vi "UI_SettingsUpdate.vi"(8 "error in (no error)":errorcluster) -> (0 "error out":errorcluster)   [LabVIEW 2020]
uses:
  Global Variables/gl_UI Ctrl Refs.vi
  Globals/gl_Calibration globals.vi
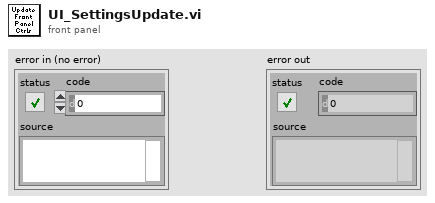
[diagram p1: front panel]
types:
  T1 = typedef "General Scan Parameters.ctl" = cluster{"Field of View":sgl, "Frame Size":u16, "Dwell Time (ms)":dbl, "Wavelength (nm)":dbl, "Zoom":dbl, "AOL Xc":sgl, "AOL Yc":sgl, "AOL Zc":sgl, "AOL Mode":enum16{"Raster", "Structural", "Pointing", "Mini Scan", "Alignment"}, "Imaging Mode":enum16{"Live Imaging", "AOL Zstack", "Motor Zstack", "Functional Imaging"}}
  T2 = typedef "UI ctrl refs cluster.ctl" = cluster{"Top level VI path":path, "Top level VI ref":refnum<vi>, "User menu ref":refnum<k9>, "Sub Panel control":refnum<vi>, "Imaging Param Tab":refnum<vi>, "Occurrence-Start drivers":refnum<k4>, "Occurrence-Speed logging initialised":refnum<k4>, "Occurrence-XYZ stage initialised":refnum<k4>, "Exit button":refnum<vi>, "Status ind":refnum<vi>, "Set as origin":refnum<vi>, "Speed Logging":refnum<vi>, "Time Lapse":refnum<vi>, "Live Imaging":refnum<vi>, "AOL Z Stack":refnum<vi>, "Motor Z Stack":refnum<vi>, "Funct Acq button":refnum<vi>, "Hard Shutter":refnum<vi>, "Virtual Shutter":refnum<vi>, "Laser Power":refnum<vi>, "AOL Mode":refnum<vi>, "Frame Size":refnum<vi>, "Field of View":refnum<vi>, "Dwell Time":refnum<vi>, "Zoom":refnum<vi>, "AOL Z":refnum<vi>, "Objective":refnum<vi>, "Axis":refnum<vi>, "Paths & Names":refnum<vi>, "Experiment folder path (ind.)":refnum<vi>, "Last State (Ind.)":refnum<vi>, "Averages":refnum<vi>, "Angle (degrees)":refnum<vi>, "X centre":refnum<vi>, "Y centre":refnum<vi>, "Plane Mode":refnum<vi>, "# Planes":refnum<vi>, "Z Start":refnum<vi>, "Z Stop":refnum<vi>, "Z Step":refnum<vi>, "PMT 1":refnum<vi>, "PMT 2":refnum<vi>, "Stage XYZ Position":refnum<vi>, "Pockels@Z Start":refnum<vi>, "Pockels@Z Stop":refnum<vi>, "Obtain Z Start":refnum<vi>, "Obtain Z Stop":refnum<vi>, "Live stim.trig.period":refnum<vi>, "Live stim.trig.enable":refnum<vi>, "Movement Correction":refnum<vi>, "Load Reference Image":refnum<vi>, "XY Stage Move":refnum<vi>, "MovCor Cluster":refnum<vi>, "RefDAQParam":refnum<vi>, "Funct. Acq. Pockels Modulation":refnum<vi>, "Ref Laser Power":refnum<vi>, "Enable Video Recording":refnum<vi>, "Video Record-Live Imaging":refnum<vi>, "Video Record-Funct acq":refnum<vi>, "Reference Source":refnum<vi>, "AOL Z-stack Chirps Ready (ind)":refnum<vi>, "Target time between mov.cor. ref triggers (ms)":refnum<vi>, "Funct. Acq. Ref frame save":refnum<vi>, "Tracking button":refnum<vi>, "Show ref plots window":refnum<vi>, "Center freq ind (nm)":refnum<vi>, "Pickup mode (ind)":refnum<vi>, "Logging queue (ind)":refnum<vi>, "Back aperture power (ind.)":refnum<vi>, "Power after objective (ind.)":refnum<vi>, "Switch user":refnum<vi>, "Ls1 Conn. Status":refnum<vi>, "Ls1Tuning Status":refnum<vi>, "Ls1 Faults":refnum<vi>, "Ls1 Connection":refnum<vi>, "Ls1 Mode":refnum<vi>, "Ls1 POWER [mW]":refnum<vi>, "Ls1Shutter":refnum<vi>, "Ls1 Wavelength":refnum<vi>, "Ls1 Note":refnum<vi>, "Ls1 Confirm Wav":refnum<vi>, "Ls1 PreChrp Prism1":refnum<vi>, "Ls1 PreChrp Prism2":refnum<vi>, "Ls1 wav top Ind":refnum<vi>, "Ls1 power top Ind":refnum<vi>, "Ls1 Pump peak Hold":refnum<vi>, "Ls1 Status Ind":refnum<vi>, "Ls1 wav cancel":refnum<vi>, "Experiment Type":refnum<vi>, "Biology Information":refnum<vi>}
  T3 = enum16{"Raster", "Structural", "Pointing", "Mini Scan", "Alignment"}
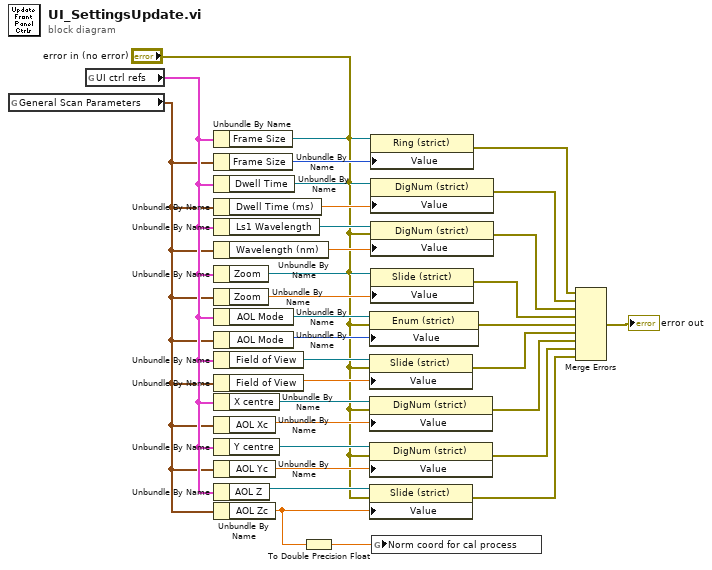
[diagram p0: block diagram]
diagram:
  n1 = global read "gl_Calibration globals.vi" "General Scan Parameters"() -> (w9:T1)
  n2 = global read "gl_UI Ctrl Refs.vi" "UI ctrl refs"() -> (w10:T2)
  n3 = Unbundle By Name(w10) -> ("Frame Size"=w32:refnum<vi>)
  n4 = Unbundle By Name(w9) -> ("Frame Size"=w31:u16)
  n5 = Unbundle By Name(w10) -> ("Dwell Time"=w29:refnum<vi>)
  n6 = Unbundle By Name(w9) -> ("Dwell Time (ms)"=w30:dbl)
  n7 = Unbundle By Name(w10) -> ("Ls1 Wavelength"=w28:refnum<vi>)
  n8 = Unbundle By Name(w9) -> ("Wavelength (nm)"=w27:dbl)
  n9 = Unbundle By Name(w10) -> ("Zoom"=w25:refnum<vi>)
  n10 = Unbundle By Name(w9) -> ("Zoom"=w26:dbl)
  n11 = Unbundle By Name(w10) -> ("AOL Mode"=w24:refnum<vi>)
  n12 = Unbundle By Name(w9) -> ("AOL Mode"=w23:T3)
  n13 = Unbundle By Name(w10) -> ("Field of View"=w21:refnum<vi>)
  n14 = Unbundle By Name(w9) -> ("Field of View"=w22:sgl)
  n15 = Unbundle By Name(w10) -> ("X centre"=w20:refnum<vi>)
  n16 = Unbundle By Name(w9) -> ("AOL Xc"=w19:sgl)
  n17 = Unbundle By Name(w10) -> ("Y centre"=w6:refnum<vi>)
  n18 = Unbundle By Name(w9) -> ("AOL Yc"=w7:sgl)
  n19 = Unbundle By Name(w10) -> ("AOL Z"=w8:refnum<vi>)
  n20 = Unbundle By Name(w9) -> ("AOL Zc"=w1:sgl)
  n21 = To Double Precision Float(number=w1) -> (double precision float=w2:dbl)
  n22 = property class="Enum (strict)"(reference=w24, error in="error in (no error)", "Value"=w23) -> (error out=w13:errorcluster)  [unwired: 1 out]
  n23 = property class="Slide (strict)"(reference=w21, error in="error in (no error)", "Value"=w22) -> (error out=w12:errorcluster)  [unwired: 1 out]
  n24 = property class="DigNum (strict)"(reference=w20, error in="error in (no error)", "Value"=w19) -> (error out=w11:errorcluster)  [unwired: 1 out]
  n25 = property class="DigNum (strict)"(reference=w6, error in="error in (no error)", "Value"=w7) -> (error out=w4:errorcluster)  [unwired: 1 out]
  n26 = property class="Slide (strict)"(reference=w8, error in="error in (no error)", "Value"=w1) -> (error out=w3:errorcluster)  [unwired: 1 out]
  n27 = property class="Ring (strict)"(reference=w32, error in="error in (no error)", "Value"=w31) -> (error out=w17:errorcluster)  [unwired: 1 out]
  n28 = property class="DigNum (strict)"(reference=w29, error in="error in (no error)", "Value"=w30) -> (error out=w16:errorcluster)  [unwired: 1 out]
  n29 = property class="DigNum (strict)"(reference=w28, error in="error in (no error)", "Value"=w27) -> (error out=w15:errorcluster)  [unwired: 1 out]
  n30 = property class="Slide (strict)"(reference=w25, error in="error in (no error)", "Value"=w26) -> (error out=w14:errorcluster)  [unwired: 1 out]
  n31 = global write "gl_Calibration globals.vi" "Norm coord for cal process"(w2) -> ()
  n32 = Merge Errors(w17, w16, w15, w14, w13, w12, w11, w4, w3) -> (→"error out":errorcluster)
